vi "WFGenD01DC.vi"(8 "error in (no error)":errorcluster, 10 "Waveform Parameters":T3) -> (0 "error out":errorcluster, 3 "Waveform Out":digitalwaveform(waveform)={"t0"=timestamp(0 s since 1904-01-01), "dt"=5e-05, "Y"={"transitions"=[], "data"=array5000x1[5000 elements]}})   [LabVIEW 2013]
uses:
  <vilib>/Waveform/DWDTOps.llb/DWDT Boolean Array to Digital.vi
  WFParameters.ctl
  WFRepetitions.ctl
panel:
  in  "WFRepetitions":T1={"Del (s)"=0.0, "Int (s)"=0.0, "N"=1} {"Int (s)" min=0.0 format="%#_4g"; "Del (s)" min=0.0 format="%#_4f"}
  in  "WFParameters":T2={"Fs (Hz)"=20000.0, "Amp (V)"=5.0, "Ramp (s)"=0.005, "Dur (s)"=0.25} {"Dur (s)" min=0.0 format="%#_4g"; "Ramp (s)" min=0.0; "Fs (Hz)" min=0.0}
  out "Digital Waveform Graph":digitalwaveform(graph)={"t0"=timestamp(0 s since 1904-01-01), "dt"=5e-05, "Y"={"transitions"=[], "data"=array5000x1[5000 elements]}}
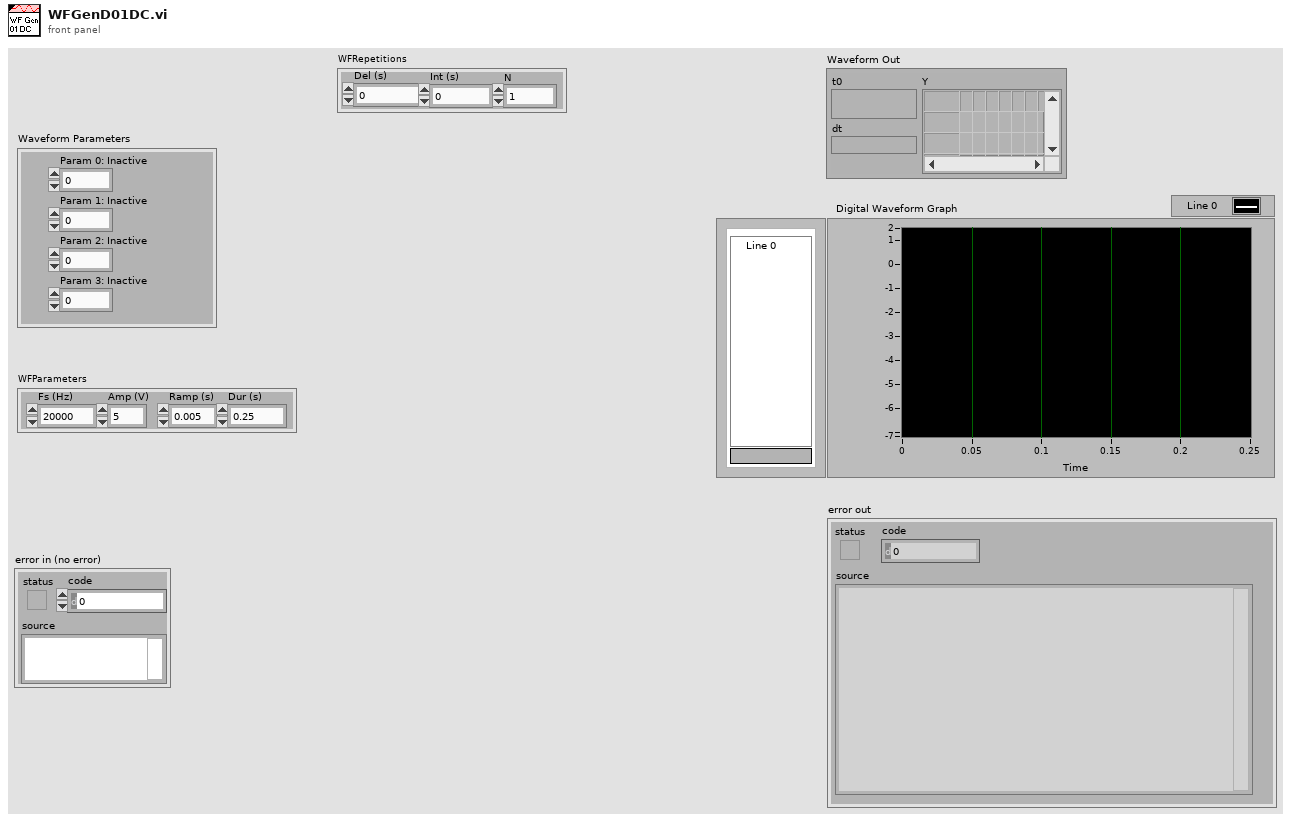
[diagram p1: front panel]
types:
  T1 = typedef "WFRepetitions.ctl" = cluster{"Del (s)":dbl, "Int (s)":dbl, "N":i32}
  T2 = typedef "WFParameters.ctl" = cluster{"Fs (Hz)":dbl, "Amp (V)":dbl, "Ramp (s)":dbl, "Dur (s)":dbl}
  T3 = cluster{"Param 0: Inactive":dbl, "Param 1: Inactive":dbl, "Param 2: Inactive":dbl, "Param 3: Inactive":dbl}
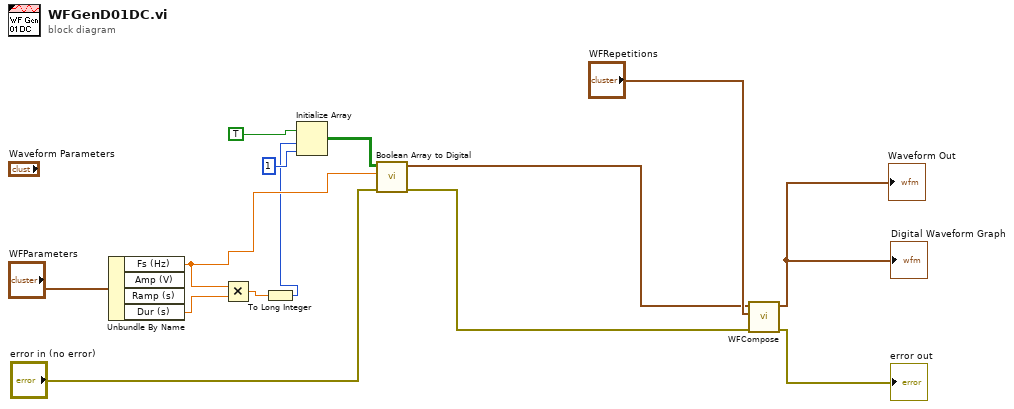
[diagram p0: block diagram]
diagram:
  n1 = Unbundle By Name("WFParameters") -> ("Fs (Hz)"=w3:dbl, "Dur (s)"=w7:dbl)  [unwired: 2 out]
  n2 = Multiply(x=w3, y=w7) -> (x*y=w2:dbl)
  n3 = To Long Integer(number=w2) -> (32bit integer=w1:i32)
  n4 = Initialize Array(TRUE, w1, 1 ("dimension size")) -> (w10:bool[][])
  n5 = call-poly <vilib>:"Boolean Array to Digital.vi"("error in (no error)"="error in (no error)", "sample rate"=w3, "boolean array"=w10) -> ("error out"=w4:errorcluster, "digital waveform"=w6:digitalwaveform)  [unwired: 7 in]
  n6 = call-poly "WFCompose.vi"("error in (no error)"=w4, "WFRepetitions"="WFRepetitions", "Waveform In"=w6) -> ("error out"=→"error out":errorcluster, "Waveform Out"=→"Waveform Out" →"Digital Waveform Graph":digitalwaveform)  [unwired: 7 in]
